vi "All Motor Controllers.vi"() -> ()   [LabVIEW 2016]
uses:
  <vilib>/Rock Robotics/SystemInterfaces/DIO/FPGA_DIOPWMChannel.ctl
  SpeedTestType.ctl
  <vilib>/Rock Robotics/WPI/ThirdParty/CanMotor/TalonSRX/WPI_CANTalonSRX_APIControlMode.ctl
  <vilib>/Rock Robotics/WPI/MotorControl/WPI_MotorControlOpen VictorSP.vi
  <vilib>/Rock Robotics/WPI/MotorControl/WPI_MotorControlOpen SPARK.vi
panel:
  in  "Speed Test Type":T1 items=["Idle", "Variable", "Full Forward", "Partial Forward", "Partial Reverse", "Full Reverse"]
  in  "Shooter motor":u8=4
  in  "Mystery motor":u8=1
  in  "Winch motor":u8=2
  in  "Collector motor":u8=3
  in  "SPARK":T2=enum."PWM 2"
  in  "Right Drive Motors":T2=enum."PWM 1"
  in  "Speed (-1 to 1)":dbl(slide) min=-1.0 max=1.0 step=0.1 scale=-1.0..1.0 scale format="%#.3f"
  in  "stop":bool
  in  "Left Drive Motors":T2
  # "Set this input before running."
  # "This can be set while running."
  # "This program requires the Driver Station to be running with Teleoperated Enabled."
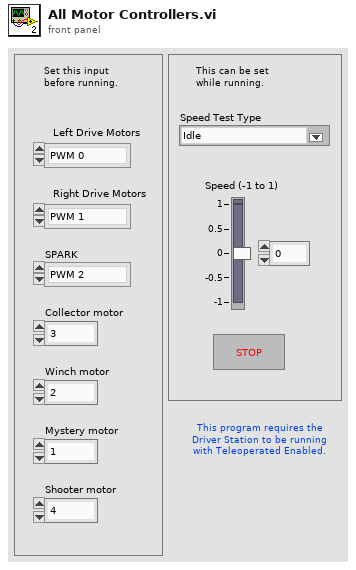
[diagram p1: front panel]
types:
  T1 = typedef "SpeedTestType.ctl" = u16
  T2 = typedef "FPGA_DIOPWMChannel.ctl" = enum8{"PWM 0", "PWM 1", "PWM 2", "PWM 3", "PWM 4", "PWM 5", "PWM 6", "PWM 7", "PWM 8", "PWM 9", "PWM MXP 0", "PWM MXP 1", "PWM MXP 2", "PWM MXP 3", "PWM MXP 4", "PWM MXP 5", "PWM MXP 6", "PWM MXP 7", "PWM MXP 8", "PWM MXP 9", "Invalid"}
  T3 = typedef "WPI_CANTalonSRX_APIControlMode.ctl" = enum8{"Percent VBus", "Speed", "Position", "Slave", "Unchanged / Invalid", "Voltage Compensation", "Current", "Motion Profile", "Motion Magic"}
  T4 = typedef "WPI_MotorControlDeviceRef.ctl" = cluster{"DeviceStatus":errorcluster, "Type":T5, "PWM":cluster{"PWM Channel":T2, "DeadBand":T6}, "CAN":cluster{"Device Number":u8, "SetOutput VI Ref":variant, "GetOutput VI Ref":variant, "Enable VI Ref":variant, "Disable VI Ref":variant, "Data":variant}, "Invert":bool}
  T5 = typedef "WPI_MotorControlType.ctl" = enum16{"PWM", "CAN"}
  T6 = typedef "WPI_PWMDeadband.ctl" = cluster{"Name":string, "maxPositivePwm":i32, "minPositivePwm":i32, "centerPwm":i32, "maxNegativePwm":i32, "minNegativePwm":i32, "angularRange":u16}
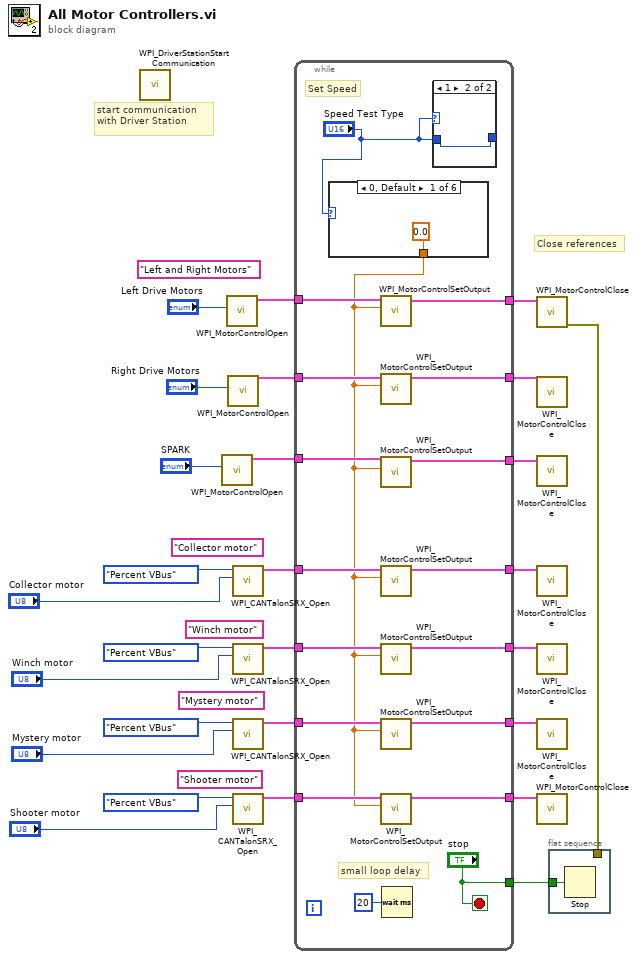
[diagram p0: block diagram]
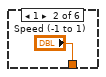
[diagram p3: hidden frame]
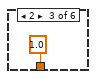
[diagram p4: hidden frame]
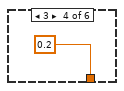
[diagram p5: hidden frame]
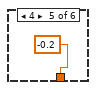
[diagram p6: hidden frame]
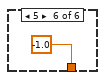
[diagram p7: hidden frame]
diagram:
  (unwired) "Left and Right Motors" ("refnum name")
  (unwired) "Shooter motor" ("refnum name")
  (unwired) "Mystery motor" ("refnum name")
  (unwired) "Winch motor" ("refnum name")
  (unwired) "Collector motor" ("refnum name")
  # "start communication with Driver Station"
  # "Close references"
  n1 = call <vilib>:"WPI_DriverStationStart Communication.vi"() -> ()  [unwired: 2 in, 10 out]
  n2 = call-poly <vilib>:"WPI_MotorControlOpen.vi"("PWM Channel"="SPARK") -> ("MotorControlDeviceRef"=w18:T4)  [unwired: 9 in, 1 out]
  n3 = call-poly <vilib>:"WPI_MotorControlOpen.vi"("PWM Channel"="Left Drive Motors") -> ("MotorControlDeviceRef"=w26:T4)  [unwired: 3 in, 7 out]
  n4 = call-poly <vilib>:"WPI_MotorControlOpen.vi"("PWM Channel"="Right Drive Motors") -> ("MotorControlDeviceRef"=w21:T4)  [unwired: 3 in, 7 out]
  n5 = call <vilib>:"WPI_CANTalonSRX_Open.vi"("Device Number"="Collector motor", "Control Mode"=WPI_CANTalonSRX_APIControlMode."Percent VBus") -> ("CAN Talon SRX Ref"=w8:T4)  [unwired: 8 in, 1 out]
  n6 = call <vilib>:"WPI_CANTalonSRX_Open.vi"("Device Number"="Winch motor", "Control Mode"=WPI_CANTalonSRX_APIControlMode."Percent VBus") -> ("CAN Talon SRX Ref"=w7:T4)  [unwired: 8 in, 1 out]
  n7 = call <vilib>:"WPI_CANTalonSRX_Open.vi"("Device Number"="Mystery motor", "Control Mode"=WPI_CANTalonSRX_APIControlMode."Percent VBus") -> ("CAN Talon SRX Ref"=w6:T4)  [unwired: 8 in, 1 out]
  n8 = call <vilib>:"WPI_CANTalonSRX_Open.vi"("Device Number"="Shooter motor", "Control Mode"=WPI_CANTalonSRX_APIControlMode."Percent VBus") -> ("CAN Talon SRX Ref"=w5:T4)  [unwired: 8 in, 1 out]
  n9 = while {
    tunnel: w26 -> [w45]
    tunnel: [w44] -> w25
    tunnel: ["stop"] -> w24
    tunnel: w21 -> [w41]
    tunnel: [w40] -> w20
    tunnel: w18 -> [w39]
    tunnel: [w38] -> w9
    tunnel: w8 -> [w37]
    tunnel: w7 -> [w36]
    tunnel: w6 -> [w35]
    tunnel: w5 -> [w34]
    tunnel: [w33] -> w4
    tunnel: [w32] -> w3
    tunnel: [w31] -> w2
    tunnel: [w30] -> w1
    stop <- "stop" stop-if-true
    # "small loop delay"
    # "Set Speed"
    n10 = case shown="0, Default" "Speed Test Type" {
      tunnel: [0.0 ("Speed (-1 to 1) 2") "Speed (-1 to 1)" 1.0 ("Speed (-1 to 1)") 0.2 ("Speed (-1 to 1)") -0.2 ("Speed (-1 to 1)") -1.0 ("Speed (-1 to 1)")] -> w29
      frame 0, Default {
      }
      frame 1 {
      }
      frame 2 {
      }
      frame 3 {
      }
      frame 4 {
      }
      frame 5 {
      }
    }
    n11 = call <vilib>:"WPI_MotorControlSetOutput.vi"("Output"=w29, "MotorControlDevRef"=w45) -> ("MotorControlDevRef"=w44:T4)  [unwired: 2 in, 7 out]
    n12 = call <vilib>:"WPI_MotorControlSetOutput.vi"("Output"=w29, "MotorControlDevRef"=w41) -> ("MotorControlDevRef"=w40:T4)  [unwired: 7 in, 2 out]
    n13 = call <vilib>:"WPI_MotorControlSetOutput.vi"("Output"=w29, "MotorControlDevRef"=w39) -> ("MotorControlDevRef"=w38:T4)  [unwired: 7 in, 2 out]
    n14 = call <vilib>:"WPI_MotorControlSetOutput.vi"("Output"=w29, "MotorControlDevRef"=w37) -> ("MotorControlDevRef"=w33:T4)  [unwired: 7 in, 2 out]
    n15 = call <vilib>:"WPI_MotorControlSetOutput.vi"("Output"=w29, "MotorControlDevRef"=w36) -> ("MotorControlDevRef"=w32:T4)  [unwired: 7 in, 2 out]
    n16 = call <vilib>:"WPI_MotorControlSetOutput.vi"("Output"=w29, "MotorControlDevRef"=w35) -> ("MotorControlDevRef"=w31:T4)  [unwired: 7 in, 2 out]
    n17 = call <vilib>:"WPI_MotorControlSetOutput.vi"("Output"=w29, "MotorControlDevRef"=w34) -> ("MotorControlDevRef"=w30:T4)  [unwired: 7 in, 2 out]
    n18 = Wait (ms)(milliseconds to wait=u32 20) -> ()  [unwired: 1 out]
    n19 = case shown="1" "Speed Test Type" {
      tunnel: [w46 w47] -> _
      tunnel: "Speed Test Type" -> [w46 w47]
      frame 0, Default {
      }
      frame 1 {
      }
    }
  }
  n20 = call <vilib>:"WPI_MotorControlClose.vi"("MotorControlDevRef"=w25) -> ("error out"=w23:errorcluster)  [unwired: 1 in, 9 out]
  n21 = call <vilib>:"WPI_MotorControlClose.vi"("MotorControlDevRef"=w20) -> ()  [unwired: 1 in, 10 out]
  n22 = call <vilib>:"WPI_MotorControlClose.vi"("MotorControlDevRef"=w9) -> ()  [unwired: 1 in, 10 out]
  n23 = call <vilib>:"WPI_MotorControlClose.vi"("MotorControlDevRef"=w4) -> ()  [unwired: 1 in, 10 out]
  n24 = call <vilib>:"WPI_MotorControlClose.vi"("MotorControlDevRef"=w3) -> ()  [unwired: 1 in, 10 out]
  n25 = call <vilib>:"WPI_MotorControlClose.vi"("MotorControlDevRef"=w2) -> ()  [unwired: 1 in, 10 out]
  n26 = call <vilib>:"WPI_MotorControlClose.vi"("MotorControlDevRef"=w1) -> ()  [unwired: 1 in, 10 out]
  n27 = flat-sequence {
    tunnel: w24 -> [w54]
    tunnel: w23 -> [_]
    frame #0 {
      n28 = Stop(stop? (T)=w54) -> ()
    }
  }
